vi "CAN-IDMenu.vi"(6 "This VI":refnum<vi>, 7 "ActIDs":sgl[](array[numeric]), 11 "_Identifier":refnum<vi>) -> ()   [LabVIEW 2016]
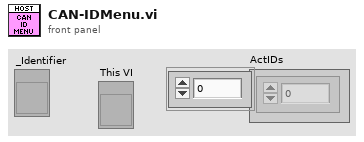
[diagram p1: front panel]
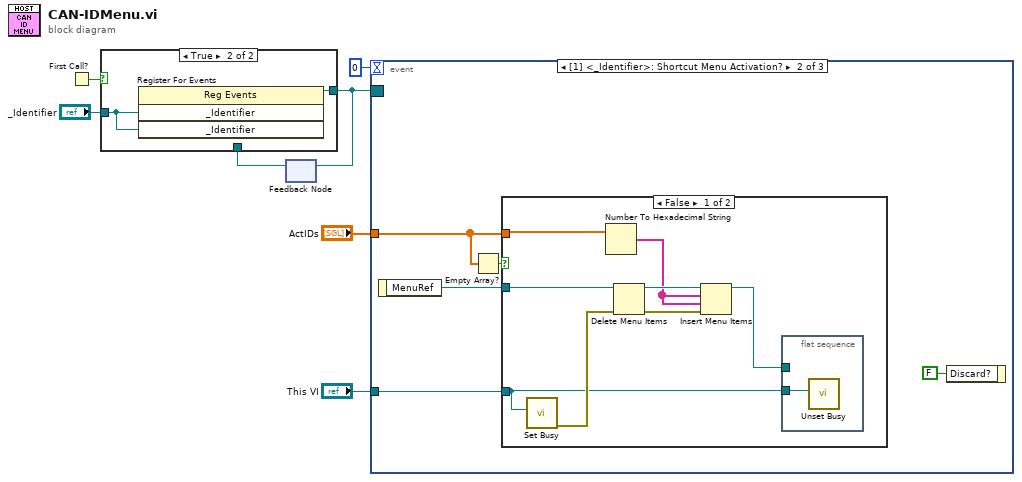
[diagram p0: block diagram]
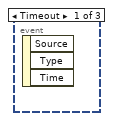
[diagram p2: hidden frame]
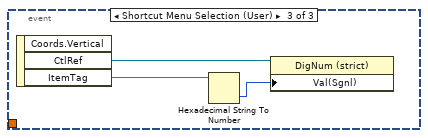
[diagram p4: hidden frame]
diagram:
  n1 = First Call?() -> (First Call?: T/F=w7:bool)
  n2 = feedback #1() -> (w5:refnum<event-registration>)  [unwired: 1 in]
  n3 = case shown="True" w7 {
    tunnel: "_Identifier" -> [_ w10]
    tunnel: [w8 w9] -> w6
    tunnel: w5 -> [w8 _]
    frame False {
    }
    frame True {
      n4 = register-events(w10, w10) -> (reference out=w9:refnum<event-registration>)  [unwired: 2 in, 1 out]
    }
  }
  n5 = feedback-in #1(w6) -> ()
  n6 = event shown="[1] <_Identifier>: Shortcut Menu Activation?" {
    selector: w6 -> [_ _ _]
    dyn-events: _ -> [_ _ _]
    timeout: 0 -> [_ _ _]
    tunnel: "ActIDs" -> [_ w11 _]
    tunnel: "This VI" -> [_ w13 _]
    event Timeout {
      n7 = event-data() -> ()  [unwired: 1 in, 3 out]
    }
    event Shortcut Menu Activation? {
      n8 = event-data() -> ("MenuRef"=w15:refnum<k9>)  [unwired: 1 in]
      n9 = Empty Array?(array=w11) -> (empty?=w12:bool)
      n10 = case shown="False" w12 {
        tunnel: w15 -> [w23 _]
        tunnel: w13 -> [w21 _]
        tunnel: w11 -> [w16 _]
        frame False {
          n11 = call <vilib>:"Set Busy.vi"("VI reference (current VI)"=w21) -> ("error out"=w22:errorcluster)  [unwired: 9 in, 1 out]
          n12 = Number To Hexadecimal String(2:w16) -> (0:w17:string[])  [unwired: 1 in]
          n13 = Delete Menu Items(6:w22, 9:w23) -> (0:w19:errorcluster, 3:w18:refnum<k9>)  [unwired: 2 in]
          n14 = Insert Menu Items(6:w19, 7:w17, 8:w17, 9:w18) -> (3:w20:refnum<k9>)  [unwired: 2 in, 2 out]
          n15 = flat-sequence {
            tunnel: w20 -> [_]
            tunnel: w21 -> [w24]
            frame #0 {
              n16 = call <vilib>:"Unset Busy.vi"("VI reference (current VI)"=w24) -> ()  [unwired: 10 in, 1 out]
            }
          }
        }
        frame True {
        }
      }
      n17 = event-data("Discard?"=FALSE) -> ()  [unwired: 1 in, 1 out]
    }
    event Shortcut Menu Selection (User) {
      n18 = event-data() -> ("CtlRef"=w27:refnum<vi>, "ItemTag"=w26:string)  [unwired: 1 in, 1 out]
      n19 = Hexadecimal String To Number(string=w26) -> (number=w25:u32)  [unwired: 2 in, 1 out]
      n20 = property class="DigNum (strict)"(reference=w27, "Val(Sgnl)"=w25) -> ()  [unwired: 1 in, 2 out]
    }
  }
